vi "Send Get Messages.vi"(7 "Message Priority (Normal)":T1=enum."Normal", 8 "error in (no error)":errorcluster, 9 "timeout in ms (-1)":i32=-1, 10 "Source":string, 11 "Message Enqueuer":refnum<class "Message Enqueuer.lvclass">) -> (0 "error out":errorcluster, 1 "timed out?":bool, 2 "Reply":variant, 3 "Message Enqueuer out":refnum<class "Message Enqueuer.lvclass">)   [LabVIEW 2024, in "Communicator Worker.lvlib" / "Get Messages Msg.lvclass"]
doc: "This VI sends the message to an actor."
uses:
  Get Messages Msg.lvclass
  Get Messages Msg.lvclass/Get Messages Msg.ctl
  C:/Program Files/National Instruments/LabVIEW 2025/vi.lib/ActorFramework/Specialty Messages/Reply Msg/Reply Msg.lvclass
  C:/Program Files/National Instruments/LabVIEW 2025/vi.lib/ActorFramework/Message/Message.lvclass
  D:/git/HAL/Source/Communicator Worker/Communicator Worker Messages/Receive Messages Msg/Get Messages Msg.lvclass
  Camera Worker/Reply Msg Generic Image Arr/Reply Msg Generic Image Arr.lvclass
  D:/git/HAL/Source/Camera Worker/Reply Msg Generic Image Arr/Reply Msg Generic Image Arr.lvclass
  <vilib>/ActorFramework/Specialty Messages/Reply Msg/Reply Msg.lvclass
  <vilib>/ActorFramework/Message Enqueuer/Message Enqueuer.lvclass
  <vilib>/ActorFramework/Message Enqueuer/Message Priority.ctl
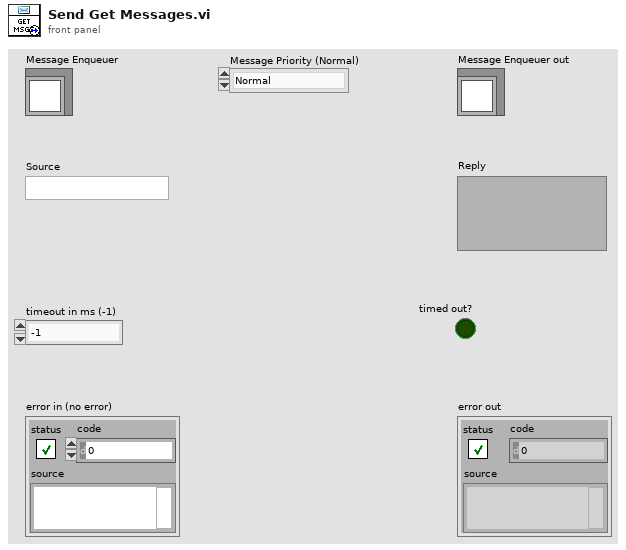
[diagram p1: front panel]
types:
  T1 = typedef "Actor Framework.lvlib/Message Enqueuer.lvclass/Message Priority.ctl" = enum16{"Low", "Normal", "High"}
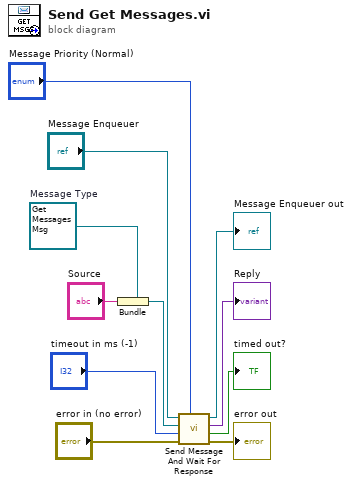
[diagram p0: block diagram]
diagram:
  w9 = refnum<class "Get Messages Msg.lvclass"> refnum  # Message Type
  n1 = Bundle(cluster=w9, "Source") -> (w8:refnum<class "Get Messages Msg.lvclass">)
  n2 = call <vilib>:"Send Message And Wait For Response.vi"("Message Priority (Normal)"="Message Priority (Normal)", "error in (no error)"="error in (no error)", "timeout in ms (-1)"="timeout in ms (-1)", "Original Message"=w8, "Message Enqueuer in"="Message Enqueuer") -> ("error out"=→"error out":errorcluster, "timed out?"=→"timed out?":bool, "Reply"=→"Reply":variant, "Message Enqueuer out"=→"Message Enqueuer out":refnum<class "Message Enqueuer.lvclass">)  [unwired: 3 in]
